vi "Update Setpoint.vi"(0 "reference in":refnum<class "HPS-17000-PowerModule.lvclass">, 11 "Error In":errorcluster) -> (4 "reference out":refnum<class "HPS-17000-PowerModule.lvclass">, 15 "Error Out":errorcluster)   [LabVIEW 2023, in "HPS-17000-PowerModule.lvlib" / "HPS-17000-PowerModule.lvclass"]
uses:
  HPS-17000-PowerModule.lvclass
  HPS-17000-PowerModule.lvclass/HPS-17000-PowerModule.ctl
  <instrlib>/HPS-17000/Internal/Write Setpoint Multi.vi
  <instrlib>/HPS-17000/HPS-17000.lvclass
  Mode.ctl
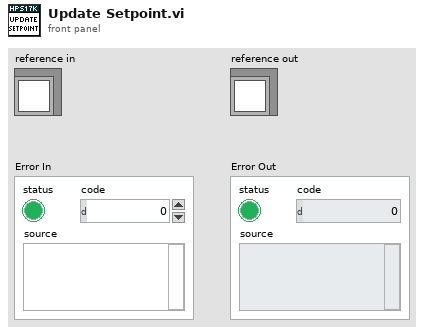
[diagram p1: front panel]
types:
  T1 = typedef "HPS-17000-PowerModule.lvlib/HPS-17000-PowerModule.lvclass/ObjectAttributes.ctl" = cluster{"JSON Config Path":path, "Configuration":T2, "GM ID":string, "HPS17000 Refs":refnum<class "HPS-17000.lvclass">[], "connected":bool, "reserved":bool, "events":T4, "nibatterycycler_grpc_Setpoint":T5, "last timestamp":i64, "mode":T6, "range":T7, "measurement array":T8[], "measurement stream":bool, "setpoint stream":bool}
  T2 = typedef "HPS-17000-PowerModule.lvlib/HPS-17000-PowerModule.lvclass/Configuration.ctl" = cluster{"TSN NIC IP Address":string, "HPS17000 IP Addresses":string[], "HPS Topology":enum16{"SINGLE", "MULTI"}, "Setpoint Stream Config":T3, "Measurement Array Size":i32}
  T3 = typedef "Cycler.lvclass/Setpoint Stream Basic Config.ctl" = cluster{"local address":string, "receiver port":u16}
  T4 = typedef "HPS-17000.lvclass/Multi-Cycler Events.ctl" = cluster{"heartbeats events":refnum<user-event>[], "faults events":refnum<user-event>[], "network sync event":refnum<user-event>[], "setpoint status event":refnum<user-event>[]}
  T5 = typedef "NI_BC_client.lvlib/nibatterycycler_grpc_Setpoint.ctl" = cluster{"voltage":sgl, "current":sgl, "min_power":sgl, "max_power":sgl, "resistance":sgl}
  T6 = typedef "HPS-17000-PowerModule.lvlib/HPS-17000-PowerModule.lvclass/Mode.ctl" = u16
  T7 = typedef "PowerModuleInterface.lvlibp/PowerModuleInterface.lvclass/Range.ctl" = cluster{"Current Max (A)":dbl, "Current Min (A)":dbl, "Voltage Max (V)":dbl, "Voltage Min (V)":dbl}
  T8 = typedef "PowerModuleInterface.lvlibp/PowerModuleInterface.lvclass/Measurements.ctl" = cluster{"measured voltage (V)":dbl, "measured current (A)":dbl, "setpoint voltage (V)":dbl, "setpoint current (A)":dbl, "timestamp":dbl}
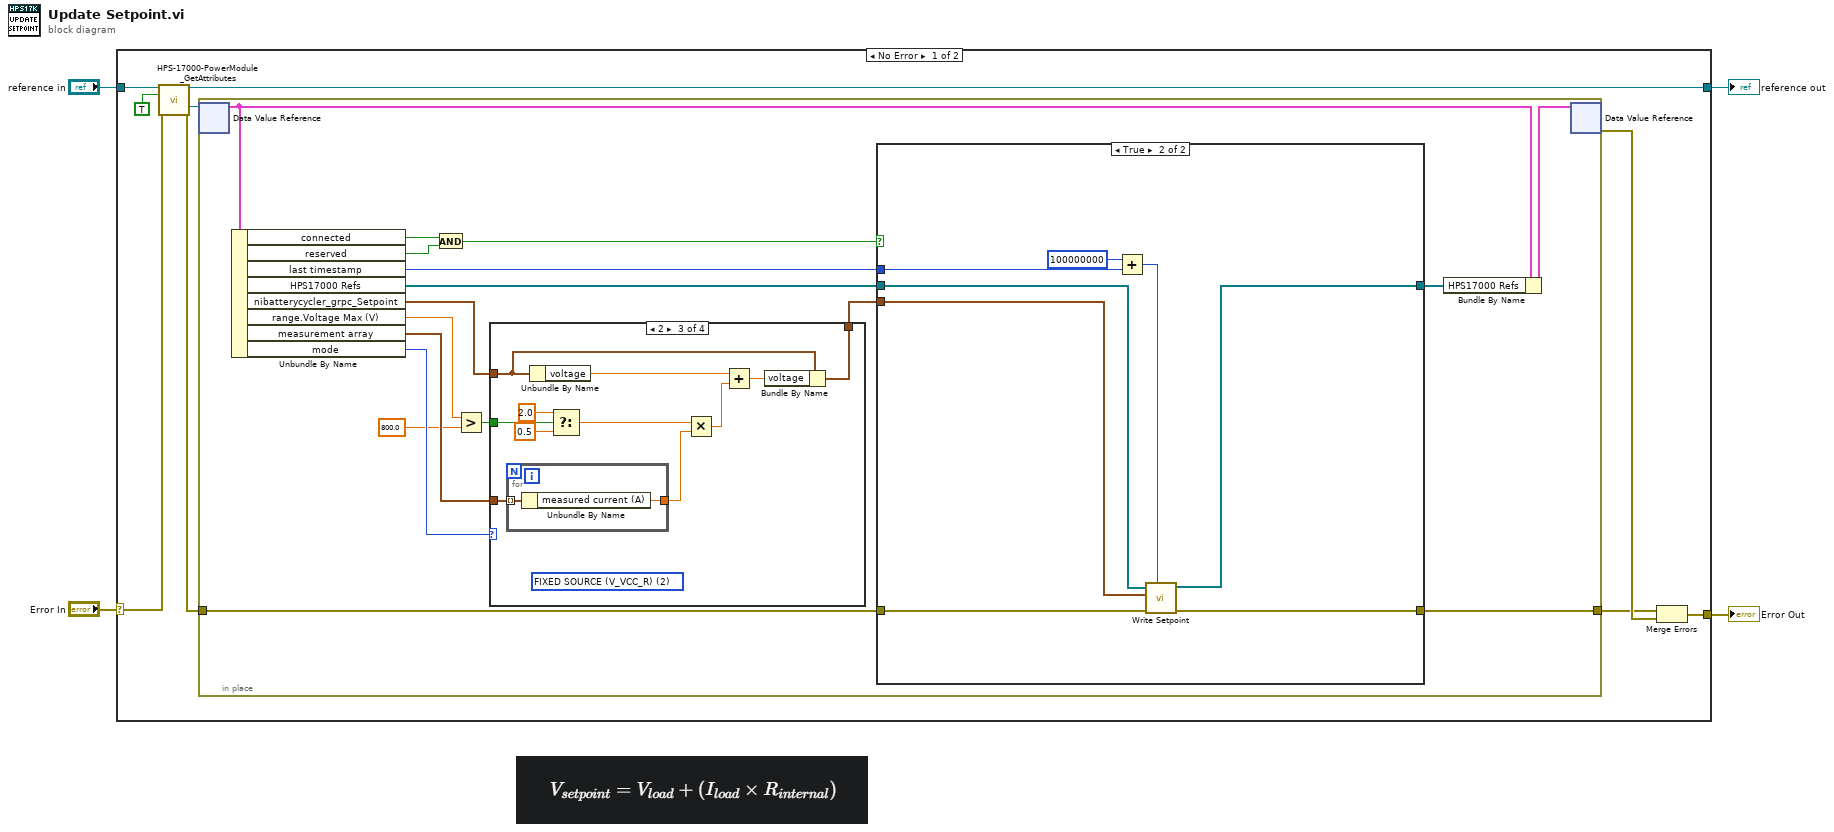
[diagram p0: block diagram]
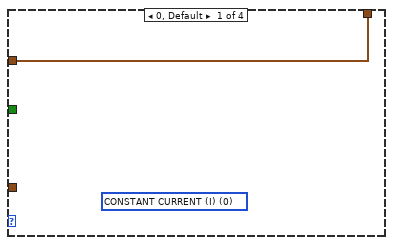
[diagram p2: hidden frame]
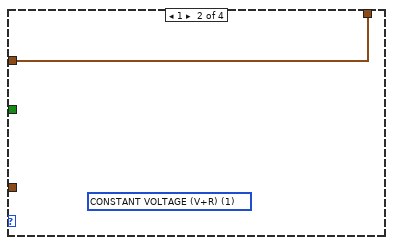
[diagram p3: hidden frame]
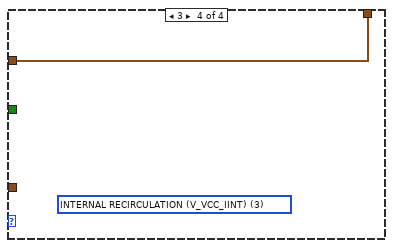
[diagram p4: hidden frame]
diagram:
  n1 = case shown="No Error" "Error In" {
    selector: "Error In" -> [w12 w58]
    tunnel: [w9 w58] -> w3
    tunnel: [w10 w57] -> w1
    tunnel: "reference in" -> [w13 w57]
    frame No Error {
      n2 = call "HPS-17000-PowerModule_GetAttributes.vi"("reference in"=w13, "OnlyGetDvrReference(False)"=TRUE, "Error In"=w12) -> ("reference out"=w10:refnum<class "HPS-17000-PowerModule.lvclass">, "DataRef"=w8:refnum<data-value>, "Error Out"=w6:errorcluster)  [unwired: 9 in, 1 out]
      n3 = in-place {
        in-place-border: w6 -> [w26]
        in-place-border: [w25] -> w5
        n4 = in-place-dvr #1(w8) -> (w29:T1)  [unwired: 1 out]
        n5 = Unbundle By Name(w29) -> ("connected"=w28:bool, "reserved"=w27:bool, "last timestamp"=w22:i64, "HPS17000 Refs"=w23:refnum<class "HPS-17000.lvclass">[], "nibatterycycler_grpc_Setpoint"=w19:T5, "range.Voltage Max (V)"=w16:dbl, "measurement array"=w17:T8[], "mode"=w20:T6)
        n6 = And(x=w28, y=w27) -> (x .and. y?=w24:bool)
        n7 = Greater?(x=w16, y=800.0) -> (0:w14:bool)
        n8 = case shown="2" w20 {
          tunnel: w17 -> [_ _ w43 _]
          tunnel: w19 -> [w31 w32 w42 w46]
          tunnel: [w31 w32 w41 w46] -> w18
          tunnel: w14 -> [_ _ w40 _]
          frame 0, Default {
            (unwired) T6 0 items=["CONSTANT CURRENT (I)", "CONSTANT VOLTAGE (V+R)", "FIXED SOURCE (V_VCC_R)", "INTERNAL RECIRCULATION (V_VCC_IINT)"] ("mode")
          }
          frame 1 {
            (unwired) T6 1 items=["CONSTANT CURRENT (I)", "CONSTANT VOLTAGE (V+R)", "FIXED SOURCE (V_VCC_R)", "INTERNAL RECIRCULATION (V_VCC_IINT)"] ("mode")
          }
          frame 2 {
            (unwired) T6 2 items=["CONSTANT CURRENT (I)", "CONSTANT VOLTAGE (V+R)", "FIXED SOURCE (V_VCC_R)", "INTERNAL RECIRCULATION (V_VCC_IINT)"] ("mode")
            n9 = for {
              tunnel: w43 -> [w45] mode=indexing
              tunnel: [w44] -> w36
              n10 = Unbundle By Name(w45) -> ("measured current (A)"=w44:dbl)
            }
            n11 = Unbundle By Name(w42) -> ("voltage"=w35:sgl)
            n12 = Select(t=2.0, s=w40, f=0.5 ("t")) -> (s? t:f=w37:dbl)
            n13 = Multiply(x=w37, y=w36) -> (x*y=w34:dbl)
            n14 = Add(x=w35, y=w34) -> (x+y=w33:dbl)
            n15 = Bundle By Name(cluster=w42, "voltage"=w33) -> (w41:T5)
          }
          frame 3 {
            (unwired) T6 3 items=["CONSTANT CURRENT (I)", "CONSTANT VOLTAGE (V+R)", "FIXED SOURCE (V_VCC_R)", "INTERNAL RECIRCULATION (V_VCC_IINT)"] ("mode")
          }
        }
        n16 = case shown="True" w24 {
          tunnel: w18 -> [_ w56]
          tunnel: w26 -> [w47 w55]
          tunnel: [w47 w54] -> w25
          tunnel: w23 -> [w48 w53]
          tunnel: w22 -> [_ w51]
          tunnel: [w48 w49] -> w21
          frame False {
          }
          frame True {
            n17 = Add(x=i64 100000000 ("y"), y=w51) -> (x+y=w50:i64)
            n18 = call-poly <instrlib>:"Write Setpoint.vi"("timestamp"=w50, "error in"=w55, "setpoint"=w56, "cycler refs in"=w53) -> ("error out"=w54:errorcluster, "cycler refs out"=w49:refnum<class "HPS-17000.lvclass">[])  [unwired: 6 in]
          }
        }
        n19 = Bundle By Name(cluster=w29, "HPS17000 Refs"=w21) -> (w30:T1)
        n20 = in-place-dvr #1(w30) -> (w11:errorcluster)  [unwired: 1 out]
      }
      n21 = Merge Errors(w5, w11) -> (w9:errorcluster)
    }
    frame Error {
    }
  }
  "Error Out" <- w3
  "reference out" <- w1
